vi "DSF.Engine.Framework.Create.Transfer Groups.vi"(8 "error in (no error)":errorcluster, 10 "Transfer Group Configurations":refnum<class "Transfer Group Configuration.lvclass">[](array[class]), 11 "Framework in":refnum<class "DSF.Engine.Framework.lvclass">) -> (0 "error out":errorcluster, 2 "Transfer Groups":refnum<class "DSF.Engine.Transfer Group.lvclass">[](array[class]), 3 "Framework out":refnum<class "DSF.Engine.Framework.lvclass">)   [LabVIEW 2017, in "Data Sharing Framework Engine.lvlib" / "DSF.Engine.Framework.lvclass"]
uses:
  DSF.Engine.Framework.lvclass
  Transfer/DSF.Engine.Transfer Group.lvclass
  Shared/Classes/Transfer Group/Transfer Group Configuration.lvclass
  DSF.Engine.Framework.lvclass/DSF.Engine.Framework.ctl
  Cache/DSF.Engine.Memory.Cache.lvclass/DSF.Engine.Memory.Cache.ctl
  Pointer/DSF.Engine.Pointer.DBL.lvclass
  C:/Program Files (x86)/National Instruments/LabVIEW 2017/vi.lib/National Instruments/Memory Manager/Classes/Pointer/Memory.Pointer.lvclass
  Shared/Classes/Transfer Group/Transfer Group Configuration.lvclass/Transfer Group Configuration.ctl
  Source/Data Sharing Framework Core/Engine/Transfer Configuration/Transfer Configuration.lvclass/Transfer Configuration.ctl
  <vilib>/National Instruments/Memory Manager/Classes/Pointer/Memory.Pointer.lvclass/Memory.Pointer.ctl
  <vilib>/National Instruments/Memory Manager/Classes/Pointer/Memory.Pointer.New.8B.vi
  <vilib>/National Instruments/Memory Manager/Classes/Pointer/Memory.Pointer.Allocate.vi
  <vilib>/National Instruments/Memory Manager/Classes/Pointer/Memory.Pointer.Set Address.vi
  <vilib>/National Instruments/Memory Manager/Classes/Pointer/Memory.Pointer.Set Size.vi
  <vilib>/National Instruments/Memory Manager/Classes/Pointer/Memory.Pointer.Set Allocated.vi
  Timing/DSF.Engine.Timing.lvclass
  Cache/DSF.Engine.Memory.Cache.lvclass
  Source/Data Sharing Framework Core/Engine/Transfer Configuration/Transfer Configuration.lvclass
  Buffer/DSF.Engine.Memory.Buffer.lvclass
  <vilib>/National Instruments/Memory Manager/Classes/Pointer/Memory.Pointer.lvclass
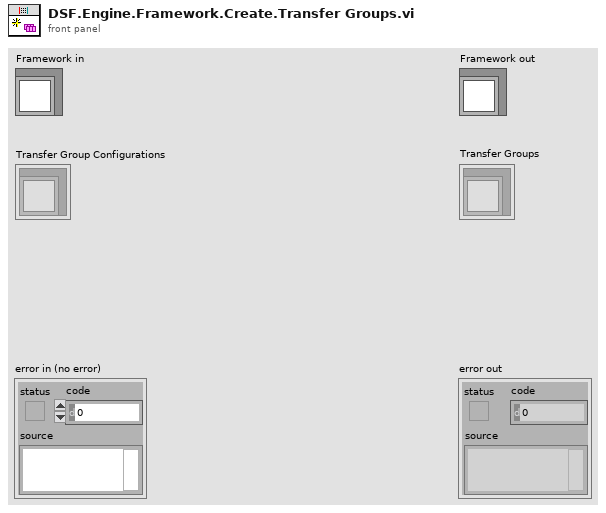
[diagram p1: front panel]
types:
  T1 = typedef "DSF Configuration API.lvlib/DSF Direction.ctl" = enum8{"Tx", "Rx"}
  T2 = typedef "DSF Configuration API.lvlib/DSF Timing Info.ctl" = cluster{"priority":u64, "decimation":u64, "offset":u64}
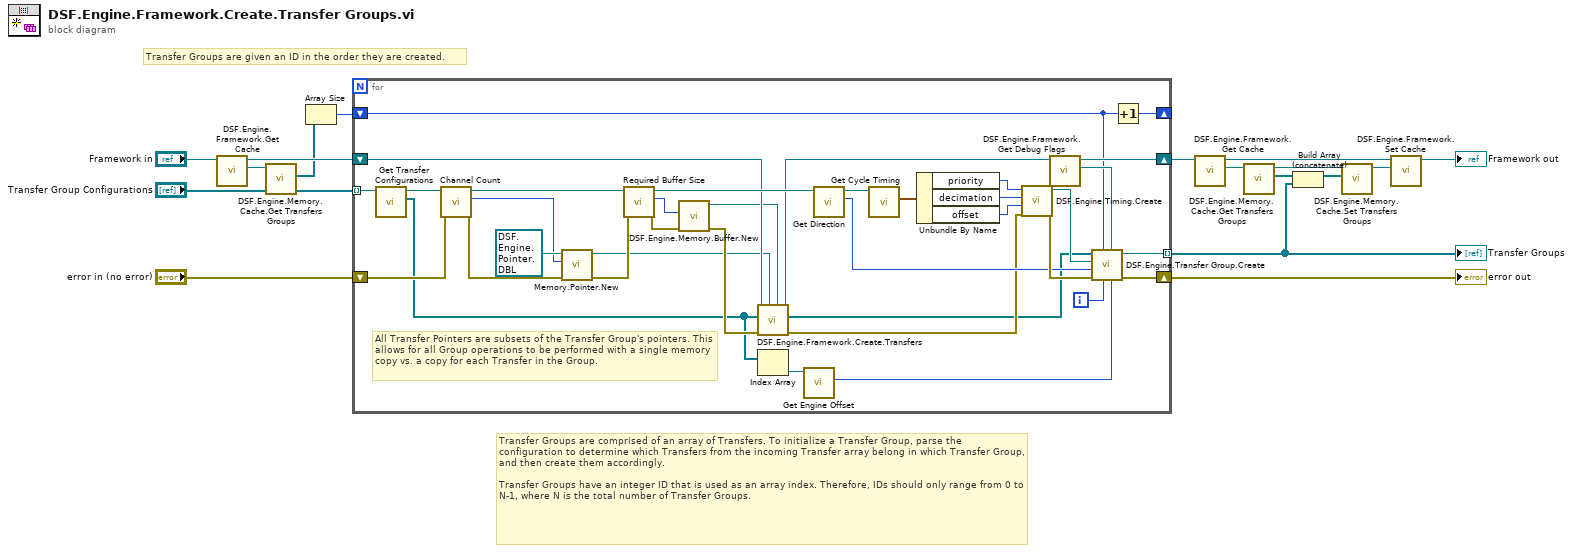
[diagram p0: block diagram]
diagram:
  # "Transfer Groups are given an ID in the order they are created."
  # "Transfer Groups are comprised of an array of Transfers. To initialize a Transfer Group, parse the configuration to determine which Transfers from the incoming Transfer array belong in which Transfer Group, and then create them accordingly.\n\nTransfer Groups have an integer ID that is used as an array index. Therefore, IDs should only range from 0 to N-1, where N is the total number of Transfer Groups."
  n1 = call "DSF.Engine.Framework.Get Cache.vi"("Framework in"="Framework in") -> ("Cache"=w6:refnum<class "DSF.Engine.Memory.Cache.lvclass">, "Framework out"=w4:refnum<class "DSF.Engine.Framework.lvclass">)  [unwired: 9 in]
  n2 = call "DSF.Engine.Memory.Cache.Get Transfers Groups.vi"("Cache in"=w6) -> ("Transfers Groups"=w3:refnum<class "DSF.Engine.Transfer Group.lvclass">[])  [unwired: 9 in, 1 out]
  n3 = Array Size(array=w3) -> (size(s)=w16:i32)
  n4 = for {
    shift-right: [w52] -> w1
    shift-left: "error in (no error)" -> [w37]
    tunnel: [w38] -> w2 mode=indexing
    shift-right: [w42] -> w8
    shift-left: w4 -> [w27]
    shift-right: [w51] -> _
    shift-left: w16 -> [w40]
    tunnel: "Transfer Group Configurations" -> [w35] mode=indexing
    i -> [w39]
    # "All Transfer Pointers are subsets of the Transfer Group's pointers. This allows for all Group operations to be performed with a single memory copy vs. a copy for each Transfer in the Group."
    n5 = call "Get Transfer Configurations.vi"("Transfer Group Configuration in"=w35) -> ("Transfer Configurations"=w20:refnum<class "Transfer Configuration.lvclass">[], "Transfer Group Configuration out"=w34:refnum<class "Transfer Group Configuration.lvclass">)  [unwired: 9 in]
    n6 = call "Channel Count.vi"("error in (no error)"=w37, "Transfer Group Configuration in"=w34) -> ("error out"=w25:errorcluster, "total channel count"=w18:u64, "Transfer Group Configuration out"=w36:refnum<class "Transfer Group Configuration.lvclass">)  [unwired: 7 in]
    n7 = call-poly <vilib>:"Memory.Pointer.New.vi"("error in (no error)"=w25, "count (1)"=w18, "Pointer type"=refnum<class "DSF.Engine.Pointer.DBL.lvclass"> refnum ("Group Intermediate Buffer")) -> ("error out"=w24:errorcluster, "Pointer"=w23:refnum<class "DSF.Engine.Pointer.DBL.lvclass">)  [unwired: 7 in]
    n8 = call "Required Buffer Size.vi"("error in (no error)"=w24, "Transfer Group Configuration in"=w36) -> ("error out"=w32:errorcluster, "required buffer size"=w33:u64, "Transfer Group Configuration out"=w53:refnum<class "Transfer Group Configuration.lvclass">)  [unwired: 7 in]
    n9 = call "DSF.Engine.Memory.Buffer.New.vi"("error in (no error)"=w32, "size"=w33) -> ("error out"=w31:errorcluster, "Buffer out"=w22:refnum<class "DSF.Engine.Memory.Buffer.lvclass">)  [unwired: 8 in]
    n10 = call "DSF.Engine.Framework.Create.Transfers.vi"("Group String Buffer"=w22, "Group Intermediate Buffer"=w23, "error in (no error)"=w31, "Transfer Configurations"=w20, "Framework in"=w27) -> ("error out"=w30:errorcluster, "Transfers"=w29:refnum<class "DSF.Engine.Transfer.lvclass">[], "Framework out"=w28:refnum<class "DSF.Engine.Framework.lvclass">)  [unwired: 4 in]
    n11 = Index Array(array=w20) -> (element=w21:refnum<class "Transfer Configuration.lvclass">)  [unwired: 1 in]
    n12 = call "Get Engine Offset.vi"("Transfer Configuration in"=w21) -> ("engine offset"=w19:u64)  [unwired: 9 in, 1 out]
    n13 = call "Get Direction.vi"("Transfer Group Configuration in"=w53) -> ("direction"=w43:T1, "Transfer Group Configuration out"=w50:refnum<class "Transfer Group Configuration.lvclass">)  [unwired: 9 in]
    n14 = call "Get Cycle Timing.vi"("Transfer Group Configuration in"=w50) -> ("cycle timing"=w49:T2)  [unwired: 9 in, 1 out]
    n15 = Unbundle By Name(w49) -> ("priority"=w45:u64, "decimation"=w46:u64, "offset"=w47:u64)
    n16 = call "DSF.Engine.Timing.Create.vi"("error in (no error)"=w30, "Offset"=w47, "Decimation"=w46, "Priority"=w45) -> ("error out"=w48:errorcluster, "Timing"=w44:refnum<class "DSF.Engine.Timing.lvclass">)  [unwired: 6 in]
    n17 = call "DSF.Engine.Framework.Get Debug Flags.vi"("Framework in"=w28) -> ("Debug Flags"=w41:refnum<class "DSF.Engine.Debug Flags.lvclass">, "Framework out"=w42:refnum<class "DSF.Engine.Framework.lvclass">)  [unwired: 9 in]
    n18 = call "DSF.Engine.Transfer Group.Create.vi"("engine offset"=w19, "Debug Flags"=w41, "transceiver id"=w39, "framework id"=w40, "error in (no error)"=w48, "Direction"=w43, "Timing"=w44, "Transfers"=w29) -> ("error out"=w52:errorcluster, "Transfer Group out"=w38:refnum<class "DSF.Engine.Transfer Group.lvclass">)  [unwired: 2 in]
    n19 = Increment(x=w40) -> (x+1=w51:i32)
  }
  "error out" <- w1
  "Transfer Groups" <- w2
  n20 = call "DSF.Engine.Framework.Get Cache.vi"("Framework in"=w8) -> ("Cache"=w13:refnum<class "DSF.Engine.Memory.Cache.lvclass">, "Framework out"=w14:refnum<class "DSF.Engine.Framework.lvclass">)  [unwired: 9 in]
  n21 = call "DSF.Engine.Memory.Cache.Get Transfers Groups.vi"("Cache in"=w13) -> ("Transfers Groups"=w10:refnum<class "DSF.Engine.Transfer Group.lvclass">[], "Cache out"=w11:refnum<class "DSF.Engine.Memory.Cache.lvclass">)  [unwired: 9 in]
  n22 = Build Array (concatenate)(w10, w2) -> (w9:refnum<class "DSF.Engine.Transfer Group.lvclass">[])
  n23 = call "DSF.Engine.Memory.Cache.Set Transfers Groups.vi"("Transfers Groups"=w9, "Cache in"=w11) -> ("Cache out"=w12:refnum<class "DSF.Engine.Memory.Cache.lvclass">)  [unwired: 9 in]
  n24 = call "DSF.Engine.Framework.Set Cache.vi"("Cache"=w12, "Framework in"=w14) -> ("Framework out"=→"Framework out":refnum<class "DSF.Engine.Framework.lvclass">)  [unwired: 9 in]
